vi "DataToStringArray.vi"(11 "MeasureData":T1) -> (3 "Array":string[](array[string]))   [LabVIEW 2013]
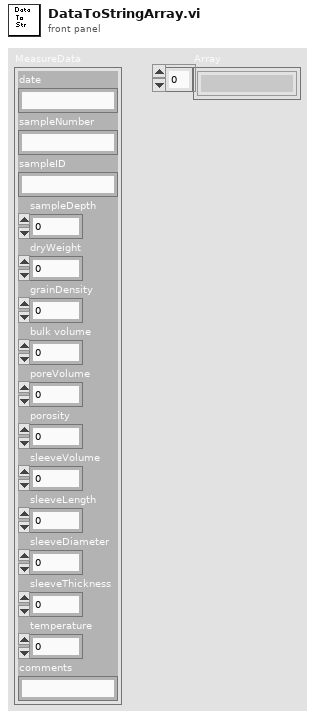
[diagram p1: front panel]
types:
  T1 = cluster{"date":string, "sampleNumber":string, "sampleID":string, "sampleDepth":dbl, "dryWeight":dbl, "grainDensity":dbl, "bulk volume":dbl, "poreVolume":dbl, "porosity":dbl, "sleeveVolume":dbl, "sleeveLength":dbl, "sleeveDiameter":dbl, "sleeveThickness":dbl, "temperature":dbl, "comments":string}
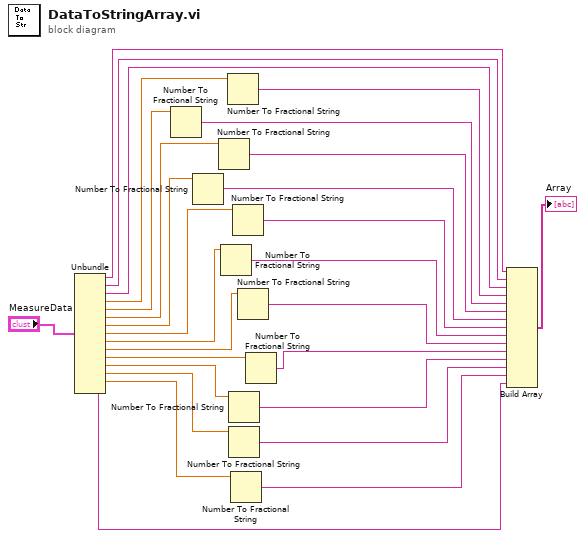
[diagram p0: block diagram]
diagram:
  n1 = Unbundle("MeasureData") -> ("date"=w1:string, "sampleNumber"=w2:string, "sampleID"=w25:string, "sampleDepth"=w22:dbl, "dryWeight"=w23:dbl, "grainDensity"=w24:dbl, "bulk volume"=w19:dbl, "poreVolume"=w17:dbl, "porosity"=w16:dbl, "sleeveVolume"=w15:dbl, "sleeveLength"=w14:dbl, "sleeveDiameter"=w13:dbl, "sleeveThickness"=w11:dbl, "temperature"=w12:dbl, "comments"=w3:string)
  n2 = Number To Fractional String(number=w23) -> (F-format string=w27:string)  [unwired: 3 in]
  n3 = Number To Fractional String(number=w19) -> (F-format string=w18:string)  [unwired: 3 in]
  n4 = Number To Fractional String(number=w24) -> (F-format string=w20:string)  [unwired: 3 in]
  n5 = Number To Fractional String(number=w16) -> (F-format string=w9:string)  [unwired: 3 in]
  n6 = Number To Fractional String(number=w22) -> (F-format string=w26:string)  [unwired: 3 in]
  n7 = Number To Fractional String(number=w13) -> (F-format string=w6:string)  [unwired: 3 in]
  n8 = Number To Fractional String(number=w11) -> (F-format string=w5:string)  [unwired: 3 in]
  n9 = Number To Fractional String(number=w12) -> (F-format string=w4:string)  [unwired: 3 in]
  n10 = Number To Fractional String(number=w17) -> (F-format string=w10:string)  [unwired: 3 in]
  n11 = Number To Fractional String(number=w15) -> (F-format string=w8:string)  [unwired: 3 in]
  n12 = Number To Fractional String(number=w14) -> (F-format string=w7:string)  [unwired: 3 in]
  n13 = Build Array(w1, w2, w25, w26, w27, w20, w18, w10, w9, w8, w7, w6, w5, w4, w3) -> (→"Array":string[])
